vi "Merge JSON Objects.vi"() -> ()   [LabVIEW 2017]
doc: "JSONtexst example showing how one can \"merge\" objects/clusters."
uses:
  6ff16e31-2e4e-4a30-b7b7-78f55a1623ad.vi
  Get all Object Items.vi
  Set Multiple Object Items.vi
  Variant to JSON Text.vi
  JSONtext.lvlib
panel:
  out "<JSON>Merged Objects (and Cluster)":string
  out "error out":errorcluster
  # "Run this VI, then see block diagram:"
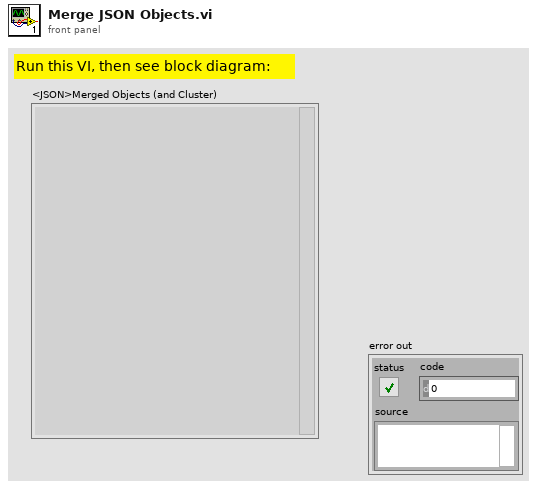
[diagram p1: front panel]
types:
  T1 = cluster{"C1":i32, "C2":string, "C3":enum16{"Enum0", "Enum1"}}
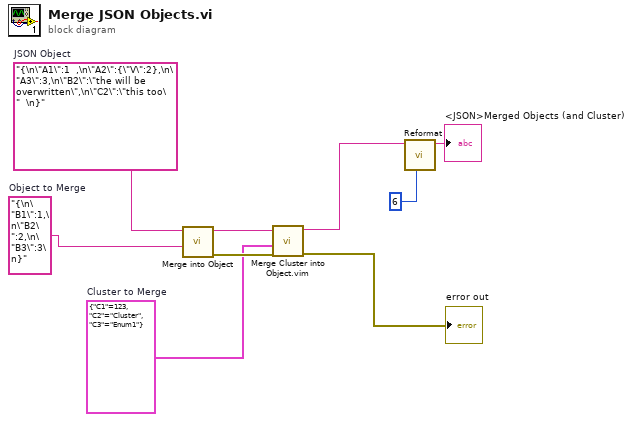
[diagram p0: block diagram]
diagram:
  w1 = T1 {"C1"=123, "C2"="Cluster", "C3"=enum."Enum1"}  # Cluster to Merge
  w8 = "{\n\"A1\":1  ,\n\"A2\":{\"V\":2},\n\"A3\":3,\n\"B2\":\"the will be overwritten\",\n\"C2\":\"this too\"  \n}"  # JSON Object
  w9 = "{\n\"B1\":1,\n\"B2\":2,\n\"B3\":3\n}"  # Object to Merge
  n1 = call "Merge into Object.vi"("Object to Merge"=w9, "JSON"=w8) -> ("error out"=w3:errorcluster, "<JSON>"=w5:string)  [unwired: 7 in]
  n2 = call "Merge Cluster into Object.vim"("error in (no error)"=w3, "Any Cluster"=w1, "JSON"=w5) -> ("error out"=→"error out":errorcluster, "<JSON>"=w4:string)  [unwired: 6 in]
  n3 = call "Reformat.vi"("Pretty Print Levels"=6, "Input String"=w4) -> ("<JSON>First JSON Value"=→"<JSON>Merged Objects (and Cluster)":string)  [unwired: 6 in, 3 out]
